vi "Main.vi"() -> ()   [LabVIEW 2016]
uses:
  <vilib>/Utility/Data Type/Type Definitions/Data Type.ctl
  <vilib>/Utility/Data Type/NI_Data Type.lvlib
panel:
  out "Type":T1
  in  "fixed-point":fxp<+/-,32,16> format="%#_21g"
  in  "LabVIEW Object":refnum<class>
  in  "Empty Refnums":T2
  in  "Complex Types":T3={"Waveform"={"t0"=timestamp(0 s since 1904-01-01), "dt"=1.0, "Y"=[]}, "Time Stamp"=timestamp(0 s since 1904-01-01), "Digital Waveform"={"t0"=timestamp(0 s since 1904-01-01), "dt"=1.0, "Y"={"transitions"=[], "data"=[]}}, "Digital Data"={"transitions"=[], "data"=[]}}
  in  "Basic Types":T4
  in  "Floats with Units":T5
  in  "Variant":variant
  in  "Enums":T6
  in  "Floats":T7
  in  "Unsigned":T8
  in  "Signed":T9
  in  "Tree":string(tree)
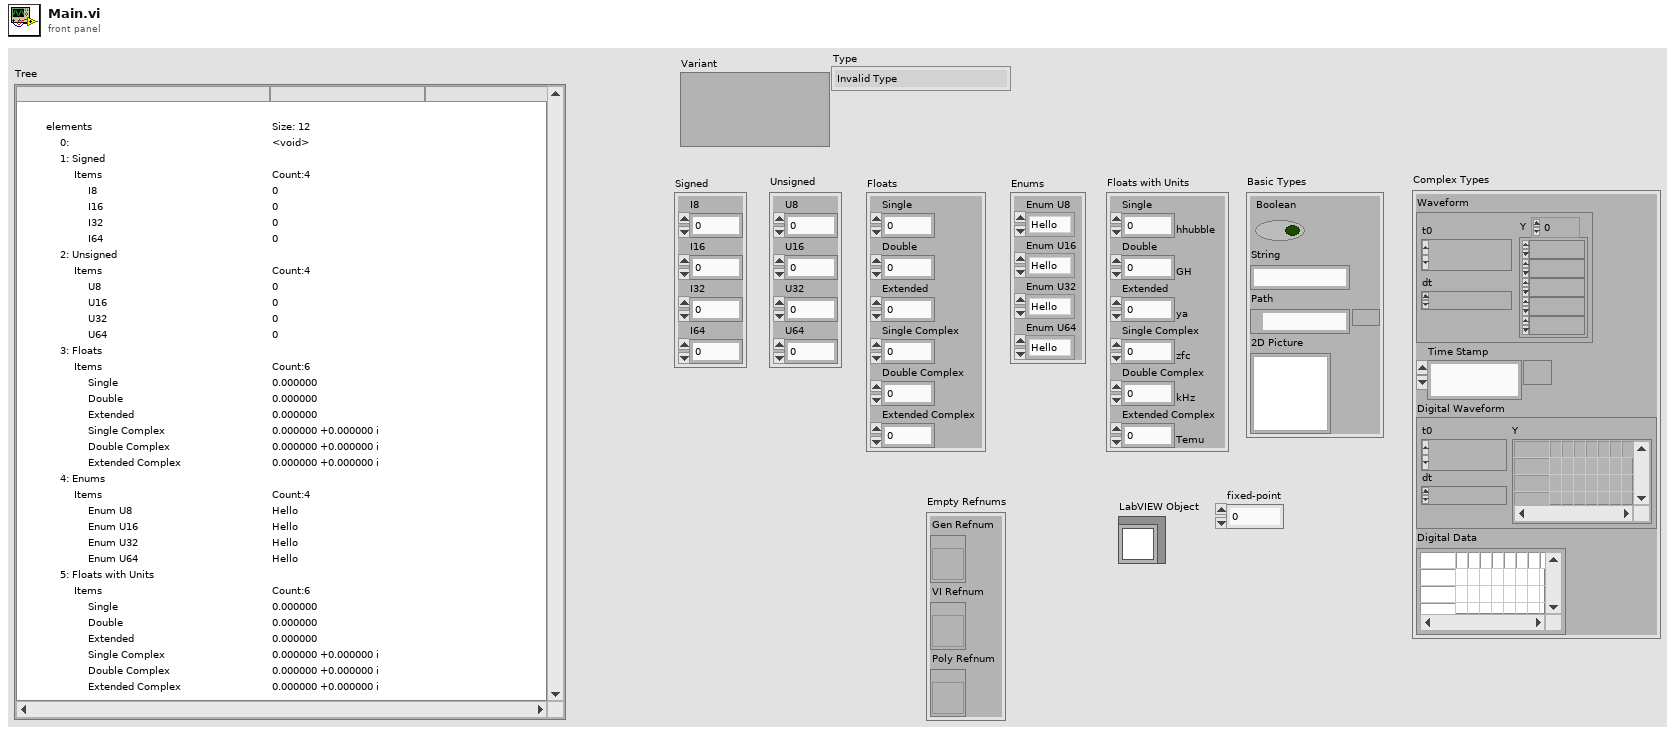
[diagram p1: front panel]
types:
  T1 = typedef "NI_Data Type.lvlib/Data Type.ctl" = enum8{"Invalid Type", "Void", "I8", "I16", "I32", "I64", "U8", "U16", "U32", "U64", "Single Float", "Double Float", "Extended Float", "Single Complex", "Double Complex", "Extended Complex", "Enum U8", "Enum U16", "Enum U32", "Enum U64", "Single Float With Unit", "Double Float With Unit", "Extended Float With Unit", "Single Complex with Unit", "Double Complex with Unit", "Extended Complex with Unit", "Boolean", "String", "Path", "Picture", "Tag", "Array", "Cluster", "Variant", "LV Variant", "Waveform", "Timestamp", "Digital Waveform", "Digital Data", "ExpressData", "Refnum", "External Data", "VI", "Poly VI", "LabVIEW Class Instance", "Fixed Point"}
  T2 = cluster{"Gen Refnum":refnum<vi>, "VI Refnum":refnum<vi>, "Poly Refnum":refnum<vi>}
  T3 = cluster{"Waveform":waveform(dbl), "Time Stamp":timestamp, "Digital Waveform":digitalwaveform, "Digital Data":digitaldata}
  T4 = cluster{"Boolean":bool, "String":string, "Path":path, "2D Picture":picture}
  T5 = cluster{"Single":sgl[unit], "Double":dbl[unit], "Extended":ext[unit], "Single Complex":csg[unit], "Double Complex":csg[unit], "Extended Complex":csg[unit]}
  T6 = cluster{"Enum U8":enum8{"Hello", "World"}, "Enum U16":enum8{"Hello", "World"}, "Enum U32":enum8{"Hello", "World"}, "Enum U64":enum8{"Hello", "World"}}
  T7 = cluster{"Single":sgl, "Double":dbl, "Extended":ext, "Single Complex":csg, "Double Complex":csg, "Extended Complex":csg}
  T8 = cluster{"U8":u8, "U16":u16, "U32":u32, "U64":u64}
  T9 = cluster{"I8":i8, "I16":i16, "I32":i32, "I64":i64}
  T10 = cluster{"Unsigned":refnum<vi>, "Variant":refnum<vi>}
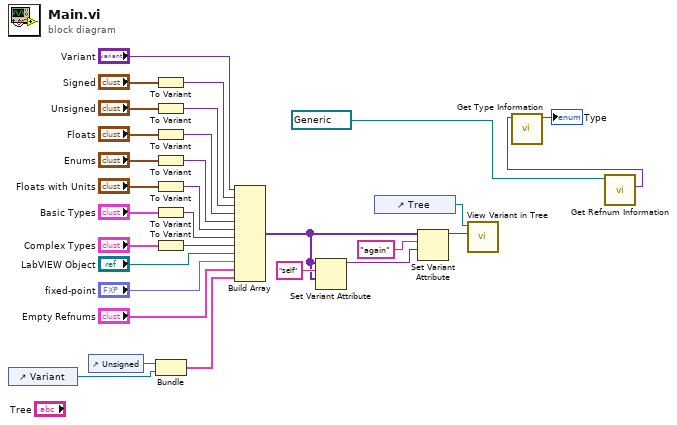
[diagram p0: block diagram]
diagram:
  n1 = control-ref of="Variant"() -> (w8:refnum<vi>)
  n2 = control-ref of="Unsigned"() -> (w6:refnum<vi>)
  n3 = To Variant(anything="Signed") -> (Variant=w26:variant)
  n4 = To Variant(anything="Unsigned") -> (Variant=w25:variant)
  n5 = To Variant(anything="Floats") -> (Variant=w24:variant)
  n6 = To Variant(anything="Enums") -> (Variant=w23:variant)
  n7 = To Variant(anything="Floats with Units") -> (Variant=w20:variant)
  n8 = To Variant(anything="Basic Types") -> (Variant=w17:variant)
  n9 = To Variant(anything="Complex Types") -> (Variant=w16:variant)
  n10 = Bundle("Unsigned"=w6, "Variant"=w8) -> (w7:T10)  [unwired: 1 in]
  n11 = Build Array("Variant", w26, w25, w24, w23, w20, w17, w16, "LabVIEW Object", "fixed-point", "Empty Refnums", w7) -> (w11:variant[])
  n12 = Set Variant Attribute(Variant=w11, name="self", value=w11) -> (Variant out=w10:variant)  [unwired: 1 in, 2 out]
  n13 = control-ref of="Tree"() -> (w30:refnum<vi>)
  n14 = Set Variant Attribute(Variant=w11, name="again", value=w10) -> (Variant out=w12:variant)  [unwired: 1 in, 2 out]
  n15 = call "View Variant in Tree.vi"("Variant"=w12, "TreeControl in"=w30) -> ()  [unwired: 9 in, 1 out]
  n16 = call <vilib>:"Get Refnum Information.vi"("Variant"=refnum<vi> refnum ("Tree")) -> ("Strict Type"=w1:variant)  [unwired: 7 in, 3 out]
  n17 = call <vilib>:"Get Type Information.vi"("Variant"=w1) -> ("Type"=→"Type":T1)  [unwired: 6 in, 4 out]
